vi "Write Multiple ELAN Values.vi"(8 "error in (no error)":errorcluster, 9 "ELAN values":T1[](array[typedef]) {"Value"."Value" format="%#_6f"}, 10 "starting address":u16, 11 "device data model in":refnum<class "ELAN Data Model.lvclass">) -> (0 "error out":errorcluster, 3 "device data model out":refnum<class "ELAN Data Model.lvclass">)   [LabVIEW 2021, in "ELAN Data Model.lvclass"]
doc: "Writes the values of multiple register values in series, starting at address M."
uses:
  ELAN Data Model.lvclass
  Type Definitions/Value full.ctl
  Data Unit/ELAN PC Data Unit/Elan units.ctl
  Data Unit/ELAN PC Data Unit/Elan measured variable.ctl
  Data Unit/ELAN PC Data Unit/Elan channel state.ctl
  ELAN Data Model.lvclass/ELAN Data Model.ctl
  Data Unit/ELAN PC Data Unit/ELAN PDU.lvclass
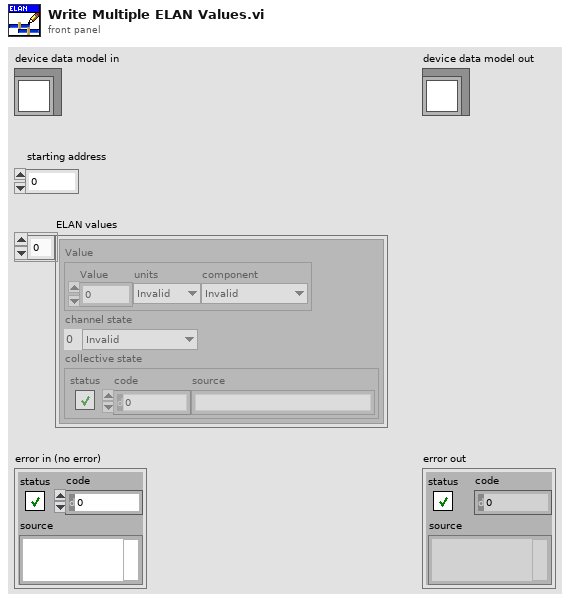
[diagram p1: front panel]
types:
  T1 = typedef "ELAN Data Model.lvclass/Value full.ctl" = cluster{"Value":cluster{"Value":sgl, "units":T2, "component":T3}, "channel state":T4, "collective state":errorcluster}
  T2 = typedef "ELAN PDU.lvclass/Elan units.ctl" = enum16{"Invalid", "no dimension", "ppm", "ppb", "vpm", "ppm C1", "ppm C3", "ppm C6", "mg C/m3", "mg/m3", "%", "% vol", "% of measuring range", "% saturation", "%/°C", "%/K", "% weight", "mV/pH", "mV/mbar", "nA/mbar", "S/m", "S/cm", "mS/m", "mS/cm", "ìS/m", "ìS/cm", "S", "min", "H", "Pa", "MA", "uV", "MV", "V", "mbar", "hPa", "Ml/min", "kOhm", "MOhm", "S1", "°C", "Hz", "pH", "ug/l", "mg/l", "l/min", "uA", "mg/dm3", "kPa", "kOhm*cm", "MOhm*cm", "°", "1/min", "1/m", "g/m3", "g/l", "% Vol C"}
  T3 = typedef "ELAN PDU.lvclass/Elan measured variable.ctl" = enum16{"Invalid", "no component", "CO", "CO2", "CH4 (Methan)", "C6H14 (Hexan)", "SO2", "NO", "NO2", "CHClF2 (R22)", "C3H8 (Propan)", "C4H10 (Butan)", "O2", "C5H12 (Pentan)", "CnHm (THC)", "P (process pressure)", "pH", "T (temperature)", "C2H4 (Ethen)", "C2H2 (Ethin)", "C3H6 (Propen)", "C4H6", "C4H8", "C2H6", "NH3 (Ammoniak)", "N2O", "C6H6 (Benzol)", "SF6", "CH3OH (Methanol)", "C2H5OH (Ethanol)", "CH2Cl2", "C2H4Cl2", "CH3Cl", "C2H4O", "H2O (water vapor)", "G/l (conductivity)", "C", "S", "N", "CF4", "COCl2 (phosgene)", "CHF3 (R23)", "C2F6 (R116)", "------ (self defined component)", "C2H3Cl", "H2 (Hydrogen)", "Ar", "He", "Cl2", "N2"}
  T4 = typedef "ELAN PDU.lvclass/Elan channel state.ctl" = enum16{"Invalid", "Warm-up", "Pause", "Standby", "Measure", "Zero calibration", "Adjust component slope", "Not yet defined1", "Adjust curve dip", "Adjust linearization sensitivity", "Adjust temperature compensation", "Adjust pressure compensation", "Adjust linearization zero", "Not yet defined2", "Autocal", "Adjust phase", "Zero calibration of O2 sensor", "Synchronous zero calibration", "Purging for synchronous zero calibration", "Adjust analog output", "Adjust analog input", "Autocal check"}
  T5 = typedef "ELAN Data Model.lvclass/Data Model.ctl" = cluster{"UTC":u64, "Value":T1[]}
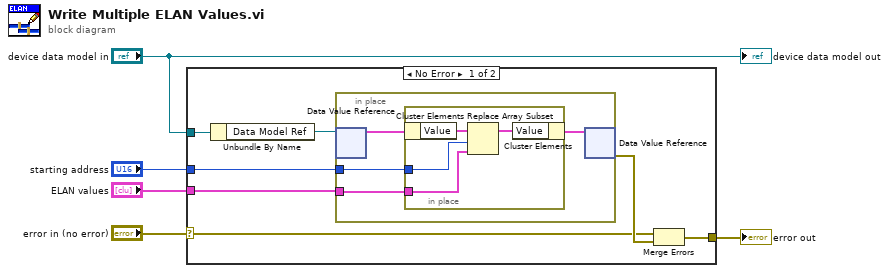
[diagram p0: block diagram]
diagram:
  n1 = case shown="No Error" "error in (no error)" {
    selector: "error in (no error)" -> [w6 w21]
    tunnel: "device data model in" -> [w12 _]
    tunnel: [w11 w21] -> w4
    tunnel: "ELAN values" -> [w10 _]
    tunnel: "starting address" -> [w9 _]
    frame No Error {
      n2 = Unbundle By Name(w12) -> ("Data Model Ref"=w8:refnum<data-value>)
      n3 = in-place {
        in-place-border: w10 -> [w16]
        in-place-border: w9 -> [w15]
        n4 = in-place-dvr #1(w8) -> (w14:T5)  [unwired: 1 out]
        n5 = in-place {
          in-place-border: w16 -> [w20]
          in-place-border: w15 -> [w19]
          n6 = in-place-cluster #2(w14) -> ("Value"=w18:T1[])
          n7 = Replace Array Subset(array=w18, new element=w20, index=w19) -> (w17:T1[])
          n8 = in-place-cluster #2("Value"=w17) -> (w13:T5)
        }
        n9 = in-place-dvr #1(w13) -> (w7:errorcluster)  [unwired: 1 out]
      }
      n10 = Merge Errors(w6, w7) -> (w11:errorcluster)
    }
    frame Error {
    }
  }
  "error out" <- w4
  "device data model out" <- "device data model in"
